vi "Profile Auton - Turn 20 Degrees Right (SubVI).vi"(8 "error in (no error)":errorcluster) -> (0 "error out":errorcluster)   [LabVIEW 2017]
uses:
  Auton Control.ctl
  <vilib>/Rock Robotics/WPI/ThirdParty/Sensors/navX/_TypeDefs/FRIC_navX_DeviceNumbersTypeDef.ctl
panel:
  in  "Cluster":T1 {"Shooting Mode" items=["No Shooter", "Low Shooter", "High Shooter"]}
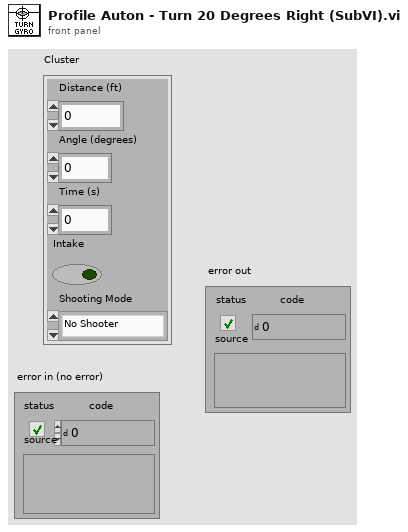
[diagram p1: front panel]
types:
  T1 = typedef "Auton Control.ctl" = cluster{"Distance (ft)":dbl, "Angle (degrees)":dbl, "Time (s)":dbl, "Intake":bool, "Shooting Mode":u16}
  T2 = typedef "FRIC_navX_DeviceNumbersTypeDef.ctl" = enum16{"Dev0", "Dev1", "Dev2", "Dev3"}
  T3 = cluster{"Yaw":dbl, "Roll":dbl, "Pitch":dbl, "Heading":dbl, "Fused Heading":dbl}
  T4 = typedef "DriveMotors.ctl" = cluster{"MotorControlDevRef":T5, "MotorControlDevRef":T5, "MotorControlDevRef":T5, "MotorControlDevRef":T5, "MotorControlDevRef":T5, "MotorControlDevRef":T5}
  T5 = typedef "WPI_MotorControlDeviceRef.ctl" = cluster{"DeviceStatus":errorcluster, "Type":T6, "PWM":cluster{"PWM Channel":T7, "DeadBand":T8}, "CAN":cluster{"Device Number":u8, "SetOutput VI Ref":variant, "GetOutput VI Ref":variant, "Enable VI Ref":variant, "Disable VI Ref":variant, "Data":variant}, "Invert":bool, "DIO PWM":cluster{"PWM \"Enable\" Channel":T7, "DIOChannel":T9, "PWM Rate":dbl}}
  T6 = typedef "WPI_MotorControlType.ctl" = enum16{"PWM", "CAN", "DIO PWM"}
  T7 = typedef "FPGA_DIOPWMChannel.ctl" = enum8{"PWM 0", "PWM 1", "PWM 2", "PWM 3", "PWM 4", "PWM 5", "PWM 6", "PWM 7", "PWM 8", "PWM 9", "PWM MXP 0", "PWM MXP 1", "PWM MXP 2", "PWM MXP 3", "PWM MXP 4", "PWM MXP 5", "PWM MXP 6", "PWM MXP 7", "PWM MXP 8", "PWM MXP 9", "Invalid"}
  T8 = typedef "WPI_PWMDeadband.ctl" = cluster{"Name":string, "maxPositivePwm":i32, "minPositivePwm":i32, "centerPwm":i32, "maxNegativePwm":i32, "minNegativePwm":i32, "angularRange":u16}
  T9 = typedef "FPGA_DIOChannel.ctl" = enum8{"DIO 0", "DIO 1", "DIO 2", "DIO 3", "DIO 4", "DIO 5", "DIO 6", "DIO 7", "DIO 8", "DIO 9", "DIO MXP 0", "DIO MXP 1", "DIO MXP 2", "DIO MXP 3", "DIO MXP 4", "DIO MXP 5", "DIO MXP 6", "DIO MXP 7", "DIO MXP 8", "DIO MXP 9", "DIO MXP 10", "DIO MXP 11", "DIO MXP 12", "DIO MXP 13", "DIO MXP 14", "DIO MXP 15", "SPI Port CS1", "SPI Port CS2", "SPI Port CS3", "SPI Port MISO", "SPI Port MOSI", "Invalid"}
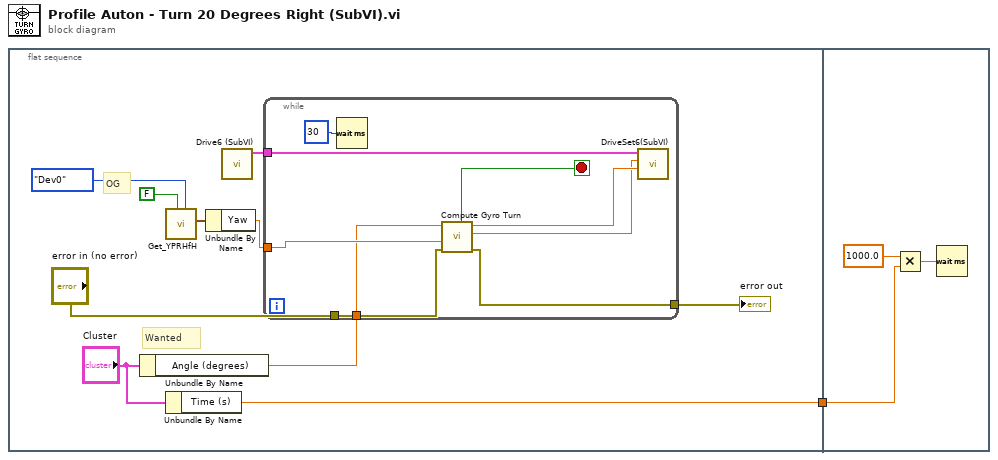
[diagram p0: block diagram]
diagram:
  n1 = flat-sequence {
    tunnel: [w2] -> w1
    tunnel: w1 -> [w21]
    frame #0 {
      # "Wanted"
      # "OG"
      n2 = Unbundle By Name("Cluster") -> ("Angle (degrees)"=w4:dbl)
      n3 = call <vilib>:"Get_YPRHfH.vi"("Device Number"=FRIC_navX_DeviceNumbersTypeDef."Dev0", "Update"=FALSE) -> ("YRPHfH"=w11:T3)  [unwired: 9 in]
      n4 = Unbundle By Name("Cluster") -> ("Time (s)"=w2:dbl)
      n5 = Unbundle By Name(w11) -> ("Yaw"=w7:dbl)
      n6 = call "Drive6 (SubVI).vi"() -> ("DriveControlDevRef"=w8:T4)  [unwired: 11 in]
      n7 = while {
        tunnel: w8 -> [w19]
        tunnel: [w14] -> w6
        tunnel: "error in (no error)" -> [w13]
        tunnel: w7 -> [w15]
        tunnel: w4 -> [w12]
        stop <- w18 stop-if-true
        n8 = Wait (ms)(milliseconds to wait=u32 30) -> ()  [unwired: 1 out]
        n9 = call "Compute Gyro Turn.vi"("error in (no error)"=w13, "Starting Degree"=w15, "Turn? Right Positive."=w12) -> ("error out"=w14:errorcluster, "Right Drive"=w16:dbl, "Left drive"=w17:dbl, "done"=w18:bool)  [unwired: 5 in]
        n10 = call "DriveSet6(SubVI).vi"("Left"=w17, "Right"=w16, "output cluster"=w19) -> ()  [unwired: 9 in]
      }
      "error out" <- w6
    }
    frame #1 {
      n11 = Multiply(x=1000.0, y=w21) -> (x*y=w23:dbl)
      n12 = Wait (ms)(milliseconds to wait=w23) -> ()  [unwired: 1 out]
    }
  }
